vi "TestExec.Script Build Return Message.vi"(3 "error in":errorcluster, 4 "Msg":T1, 5 "Data1":variant) -> (0 "error out":errorcluster, 2 "RetStr":string)   [LabVIEW 2017]
uses:
  Controls/TestExec.Script Message.ctl
panel:
  # "Data2 = Seq# and Data Error\nData1 = Data"
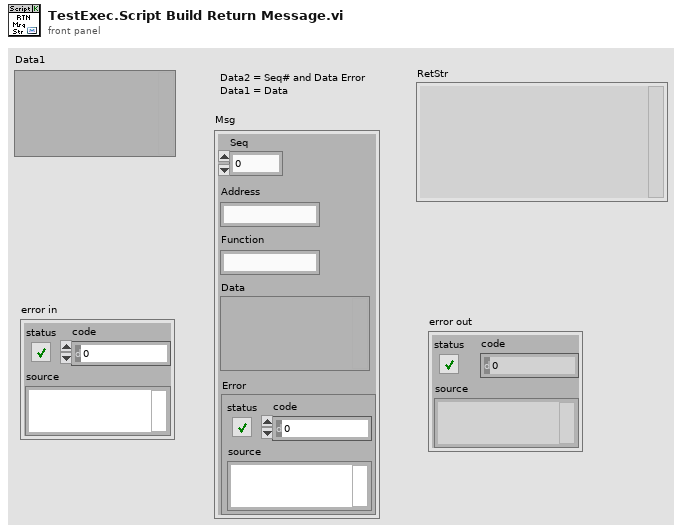
[diagram p1: front panel]
types:
  T1 = typedef "TestExec.Script Message.ctl" = cluster{"Seq":i32, "Address":string, "Function":string, "Data":variant, "Error":errorcluster}
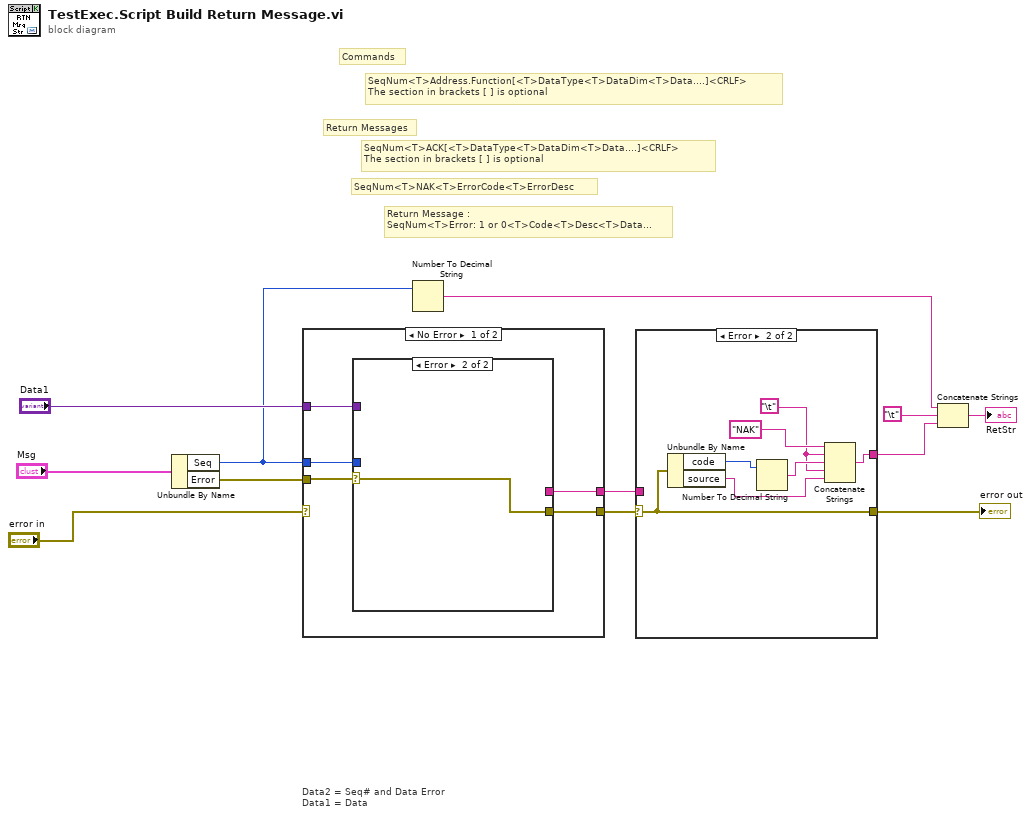
[diagram p0: block diagram]
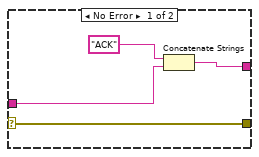
[diagram p2: hidden frame]
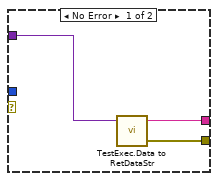
[diagram p3: hidden frame]
diagram:
  # "Return Messages"
  # "Commands"
  # "SeqNum<T>NAK<T>ErrorCode<T>ErrorDesc"
  # "SeqNum<T>ACK[<T>DataType<T>DataDim<T>Data....]<CRLF>  \nThe section in brackets [ ] is optional"
  # "SeqNum<T>Address.Function[<T>DataType<T>DataDim<T>Data....]<CRLF>\nThe section in brackets [ ] is optional"
  # "Return Message :\nSeqNum<T>Error: 1 or 0<T>Code<T>Desc<T>Data..."
  # "Data2 = Seq# and Data Error\nData1 = Data"
  n1 = Unbundle By Name("Msg") -> ("Seq"=w10:i32, "Error"=w11:errorcluster)
  n2 = case shown="No Error" "error in" {
    selector: "error in" -> [_ w22]
    tunnel: "Data1" -> [w17 _]
    tunnel: w11 -> [w16 _]
    tunnel: [w15 w22] -> w8
    tunnel: w10 -> [w14 _]
    tunnel: [w13 _] -> w7
    frame No Error {
      n3 = case shown="Error" w16 {
        selector: w16 -> [_ w21]
        tunnel: w17 -> [w20 _]
        tunnel: [w19 w21] -> w15
        tunnel: w14 -> [_ _]
        tunnel: [w18 _] -> w13
        frame No Error {
          n4 = call "TestExec.Data to RetDataStr.vi"("Data"=w20) -> ("error out"=w19:errorcluster, "RetStr"=w18:string)  [unwired: 3 in]
        }
        frame Error {
        }
      }
    }
    frame Error {
    }
  }
  n5 = Number To Decimal String(number=w10) -> (decimal integer string=w9:string)  [unwired: 1 in]
  n6 = case shown="Error" w8 {
    selector: w8 -> [w23 w31]
    tunnel: w7 -> [w25 _]
    tunnel: [w24 w27] -> w6
    tunnel: [w23 w31] -> w4
    frame No Error {
      n7 = Concatenate Strings("ACK", w25) -> (w24:string)
    }
    frame Error {
      w29 = "\t"
      n8 = Unbundle By Name(w31) -> ("code"=w32:i32, "source"=w28:string)
      n9 = Number To Decimal String(number=w32) -> (decimal integer string=w30:string)  [unwired: 1 in]
      n10 = Concatenate Strings("NAK", w29, w30, w29, w28) -> (w27:string)
    }
  }
  "error out" <- w4
  n11 = Concatenate Strings(w9, "\t", w6) -> (→"RetStr":string)
